vi "UHR-Fleezers Control (host) - Lorentz v5.vi"() -> ()   [LabVIEW 2014] (continued)
  n60 = Bundle("New Image"=w49, "New Image"=w48, "New Image"=w31, "New Image"=w47, "New Image"=w46) -> (w45:T34)  [unwired: 1 in]
  n61 = xnode "Open FPGA VI Reference"("resource name"=T27 "RIO0") -> ("FPGA VI Reference Out"=w26:T35, "error out"=w25:errorcluster)  [unwired: 1 in]
  n62 = xnode "Invoke Method"("FPGA VI Reference In"=w26, "error in"=w25) -> ("FPGA VI Reference Out"=w6:T35, "error out"=→"FPGA error out":errorcluster)
  n63 = Subtract(x=w4, y="Maximum Delta\n(MHz)") -> (x-y=w2:dbl)
  n64 = Bundle By Name(cluster=T23 {"Minimum"=60.0, "Maximum"=90.0, "Increment"=1.0} ("Min Max Inc"), "Minimum"=w2, "Maximum"=w4) -> (w1:T23)
  n65 = node-c288() -> (w52:T36)  [unwired: 4 in]
  n66 = timed-loop "Run Scripts, including: stage motion" {
    tunnel: w55 -> [w218]
    tunnel: w9 -> [w219]
    tunnel: [w219] -> w54
    tunnel: [w218] -> w53
    timing: w52 -> [_]
    timing-out: [_] -> w51
    tunnel: w43 -> [w217]
    tunnel: w44 -> [w216]
    tunnel: w39 -> [w213]
    tunnel: w38 -> [w212]
    tunnel: w37 -> [w214]
    tunnel: w36 -> [w215]
    tunnel: w28 -> [w211]
    tunnel: w21 -> [w210]
    tunnel: w8 -> [w209]
    tunnel: w7 -> [w208]
    stop <- w220 stop-if-true
    n67 = node-c288() -> ()  [unwired: 1 in, 1 out]
    n68 = event shown="[17] \"Got Bead 1\": Value Change" {
      selector: _ -> [_ _ _ _ _ _ _ _ _ _ _ _ _ _ _ _ _ _ _ _ _ _ _ _ _ _ _ _]
      dyn-events: _ -> [_ _ _ _ _ _ _ _ _ _ _ _ _ _ _ _ _ _ _ _ _ _ _ _ _ _ _ _]
      timeout: _ -> [_ _ _ _ _ _ _ _ _ _ _ _ _ _ _ _ _ _ _ _ _ _ _ _ _ _ _ _]
      tunnel: ["Set Position" "Move to Position" _ _ _ _ _ _ "Read Harvard" _ _ _ _ _ _ _ _ "Got Bead 1" "Force FB Data\nScript" _ "Got Bead 2" _ "Take Stepping Data" _ "Take Detection Laser\nImage" _ _ _] -> _
      tunnel: [_ _ _ _ _ _ _ _ _ _ _ _ _ _ _ _ _ _ _ _ _ _ _ _ _ _ w1147 _] -> w220
      tunnel: w218 -> [w239 w247 w260 w290 _ _ _ _ _ w427 w461 w487 w519 w608 w637 w769 w796 _ w838 _ _ _ _ _ _ _ _ _]
      tunnel: w219 -> [w240 w248 w261 w291 _ _ _ _ _ w428 w462 w488 w520 w609 w638 w770 w797 _ w839 _ _ _ _ _ _ _ _ _]
      tunnel: w217 -> [_ _ _ _ _ _ _ _ w412 _ _ _ _ _ _ _ _ _ _ _ _ _ _ _ _ _ _ _]
      tunnel: w216 -> [_ _ _ _ _ _ _ _ w411 _ _ _ _ _ _ _ _ _ _ _ _ _ _ _ _ _ _ _]
      tunnel: w215 -> [_ _ _ _ _ _ _ _ _ _ _ _ _ _ _ _ _ _ _ _ _ _ _ _ _ _ _ _]
      tunnel: w214 -> [_ _ _ _ _ _ _ _ _ _ _ _ _ _ _ _ _ _ _ _ _ _ _ _ _ _ _ _]
      tunnel: w213 -> [_ _ _ _ _ _ _ _ _ _ _ _ _ _ _ _ _ _ _ _ _ _ _ _ _ _ _ _]
      tunnel: w212 -> [_ _ _ _ _ _ _ _ _ _ _ _ _ _ _ _ _ _ _ _ _ _ _ _ _ _ _ _]
      tunnel: w211 -> [_ _ _ _ w318 w325 w353 w372 _ _ _ _ _ _ _ _ _ _ _ _ _ _ _ _ _ _ w1146 _]
      tunnel: w210 -> [_ _ _ _ _ _ _ _ _ _ _ _ _ _ _ _ _ _ _ _ _ _ _ _ _ w1013 _ _]
      tunnel: w209 -> [_ _ _ _ _ _ _ _ _ _ _ _ _ _ _ _ _ _ _ _ _ _ _ _ _ _ _ w1157]
      tunnel: w208 -> [_ _ _ _ _ _ _ _ _ _ _ _ _ _ _ _ _ _ _ _ _ _ _ _ _ _ _ w1152]
      tunnel: [_ _ _ _ _ _ _ _ _ _ _ _ _ _ _ _ _ _ _ _ _ "Get New Beads" _ _ _ _ _ _] -> _
      event "Set Position", "Set Position 2", "Set Position 3", "Set Position 4", "Set Position 5", "Set Position 1", "Set Position 6": Value Change {
        n69 = event-data() -> ()  [unwired: 1 in, 5 out]
        n70 = Build Array("Set Position 1", "Set Position 2", "Set Position 3", "Set Position 4", "Set Position 5", "Set Position 6") -> (w238:bool[])
        n71 = Boolean Array To Number(Boolean array=w238) -> (number=w237:u32)
        n72 = Logarithm Base 2(1:w237) -> (0:w229:dbl)
        n73 = call "Read Stage Position.vi"("error in"=w239, "VISA resource name in"=w240) -> ("Current Position"=w244:cluster{dbl, dbl, dbl}, "error out"=w243:errorcluster)  [unwired: 2 out]
        n74 = Decrement(x="Position") -> (x-1=w227:dbl)
        n75 = Greater Or Equal?(x=w229, y=0.0) -> (x >= y?=w230:bool)
        n76 = Cluster To Array(cluster=w244) -> (array=w241:dbl[])
        n77 = local write "Stage Control Serial Error"(w243) -> ()
        n78 = Select(t=w229, s=w230, f=w227) -> (s? t:f=w226:dbl)
        n79 = Increment(x=w226) -> (x+1=w225:dbl)
        n80 = Build Array (concatenate)(w225, w241) -> (w224:dbl[])
        n81 = Replace Array Subset(array="Saved Stage Positions", new element=w224, index (row)=w226) -> (w242:dbl[][])  [unwired: 1 in]
        n82 = local write "Saved Stage Positions"(w242) -> ()
      }
      event "Move to Position": Value Change {
        n83 = event-data() -> ()  [unwired: 1 in, 5 out]
        n84 = flat-sequence {
          tunnel: w248 -> [w252]
          tunnel: w247 -> [w251]
          frame #0 {
            n85 = local read "Saved Stage Positions"() -> (w254:dbl[][])
            n86 = local read "Position"() -> (w253:dbl)
            n87 = local write "Stage Moving"(TRUE ("Stage Moving")) -> ()
            n88 = call "move to saved stage position.vi"("error in"=w251, "Stage VISA resource name in"=w252, "Position"=w253, "Saved Stage Positions"=w254) -> ("error out"=w250:errorcluster)  [unwired: 1 out]
            n89 = local write "Stage Control Serial Error"(w250) -> ()
          }
          frame #1 {
            n90 = call <vilib>:"Beep.vi"() -> ()  [unwired: 3 in, 9 out]
            n91 = local write "Stage Moving"(FALSE ("Stage Moving")) -> ()
          }
        }
      }
      event "Move Cap. 1 (DNA Bottom)": Value Change {
        n92 = event-data() -> ()  [unwired: 1 in, 5 out]
        n93 = local write "Move Cap. 1 (DNA Bottom)"(FALSE ("Move Cap. 1 (DNA Right)")) -> ()
        n94 = flat-sequence {
          tunnel: w260 -> [w263]
          tunnel: w261 -> [w264]
          tunnel: [w264] -> w258
          tunnel: [w263] -> w257
          tunnel: w258 -> [w266]
          tunnel: w257 -> [w265]
          frame #0 {
            n95 = property on="Sample Channel\nFlow" class="Bool (strict)"("Val(Sgnl)"="Cap 1 Samp Flow ON") -> ()  [unwired: 2 in, 2 out]
          }
          frame #1 {
            n96 = local read "Saved Stage Positions"() -> (w276:dbl[][])
            n97 = local write "Stage Moving"(TRUE ("Stage Moving")) -> ()
            n98 = Array Subset(array=w276, index (row)=0 ("index"), length (row)=1 ("length"), index (col)=1 ("index"), length (col)=3 ("length")) -> (w273:dbl[][])
            n99 = Reshape Array(w273, 3 ("dimension size")) -> (w271:dbl[])
            n100 = Array To Cluster(array=w271) -> (cluster=w270:cluster{"[0]":dbl, "[1]":dbl, "[2]":dbl})
            n101 = call "Set Stage Position.vi"("Position"=w270, "error in"=w265, "VISA resource name in"=w266) -> ("error out"=w269:errorcluster)  [unwired: 2 out]
            n102 = local write "Stage Control Serial Error"(w269) -> ()
          }
          frame #2 {
            n103 = local write "Stage Moving"(FALSE ("Stage Moving")) -> ()
            n104 = case shown="True" "Cap 1 Flow ON" {
              frame False {
              }
              frame True {
                n105 = property on="Inject Pump 1" class="Bool (strict)"("Val(Sgnl)"=TRUE ("Value (Signaling)")) -> ()  [unwired: 2 in, 2 out]
              }
            }
            n106 = call <vilib>:"Beep.vi"() -> ()  [unwired: 3 in, 9 out]
          }
          frame #3 {
            n107 = property on="Sample Channel\nFlow" class="Bool (strict)"("Val(Sgnl)"=FALSE ("Value (Signaling)")) -> ()  [unwired: 2 in, 2 out]
            n108 = local read "Cap. 2 BD T1?\n(ADig T1, DNA T2)"() -> (w283:bool)
            n109 = case shown="True" w283 {
              tunnel: "Cap 1 T ON" -> [w285 w286]
              frame False {
                n110 = property on="Trap 1 (ON/OFF)" class="Bool (strict)"("Val(Sgnl)"=w285) -> ()  [unwired: 2 in, 2 out]
              }
              frame True {
                n111 = property on="Trap 2 (ON/OFF)" class="Bool (strict)"("Val(Sgnl)"=w286) -> ()  [unwired: 2 in, 2 out]
              }
            }
            n112 = property on="Got Bead 2" class="Bool"("Key Focus"=TRUE) -> ()  [unwired: 2 in, 2 out]
          }
        }
      }
      event "Move Cap. 2 (ADig Top)": Value Change {
        n113 = event-data() -> ()  [unwired: 1 in, 5 out]
        n114 = local write "Move Cap. 2 (ADig Top)"(FALSE ("Move Cap. 2 (ADig Left)")) -> ()
        n115 = flat-sequence {
          tunnel: w290 -> [w293]
          tunnel: w291 -> [w294]
          tunnel: [w294] -> w288
          tunnel: [w293] -> w287
          tunnel: w288 -> [w297]
          tunnel: w287 -> [w296]
          frame #0 {
            n116 = property on="Sample Channel\nFlow" class="Bool (strict)"("Val(Sgnl)"="Cap 2 Samp Flow ON") -> ()  [unwired: 2 in, 2 out]
          }
          frame #1 {
            w295 = FALSE ("Value (Signaling)")
            n117 = local read "Saved Stage Positions"() -> (w307:dbl[][])
            n118 = local write "Stage Moving"(TRUE ("Stage Moving")) -> ()
            n119 = Array Subset(array=w307, index (row)=1 ("index"), length (row)=1 ("length"), index (col)=1 ("index"), length (col)=3 ("length")) -> (w304:dbl[][])
            n120 = Reshape Array(w304, 3 ("dimension size")) -> (w302:dbl[])
            n121 = property on="Trap 1 (ON/OFF)" class="Bool (strict)"("Val(Sgnl)"=w295) -> ()  [unwired: 2 in, 2 out]
            n122 = property on="Trap 1 (ON/OFF)" class="Bool (strict)"("Val(Sgnl)"=w295) -> ()  [unwired: 2 in, 2 out]
            n123 = Array To Cluster(array=w302) -> (cluster=w301:cluster{"[0]":dbl, "[1]":dbl, "[2]":dbl})
            n124 = call "Set Stage Position.vi"("Position"=w301, "error in"=w296, "VISA resource name in"=w297) -> ("error out"=w300:errorcluster)  [unwired: 2 out]
            n125 = local write "Stage Control Serial Error"(w300) -> ()
          }
          frame #2 {
            n126 = local write "Stage Moving"(FALSE ("Stage Moving")) -> ()
            n127 = call <vilib>:"Beep.vi"() -> ()  [unwired: 3 in, 9 out]
            n128 = case shown="True" "Cap 2 Flow ON" {
              frame False {
              }
              frame True {
                n129 = property on="Inject Pump 3" class="Bool (strict)"("Val(Sgnl)"=TRUE ("Value (Signaling)")) -> ()  [unwired: 2 in, 2 out]
              }
            }
          }
          frame #3 {
            n130 = property on="Sample Channel\nFlow" class="Bool (strict)"("Val(Sgnl)"=FALSE ("Value (Signaling)")) -> ()  [unwired: 2 in, 2 out]
            n131 = case shown="False" "Cap. 2 BD T1?\n(ADig T1, DNA T2)" {
              tunnel: "Cap 2 T ON" -> [w316 w317]
              frame False {
                n132 = property on="Trap 2 (ON/OFF)" class="Bool (strict)"("Val(Sgnl)"=w316) -> ()  [unwired: 2 in, 2 out]
              }
              frame True {
                n133 = property on="Trap 1 (ON/OFF)" class="Bool (strict)"("Val(Sgnl)"=w317) -> ()  [unwired: 2 in, 2 out]
              }
            }
            n134 = property on="Got Bead 1" class="Bool"("Key Focus"=TRUE) -> ()  [unwired: 2 in, 2 out]
          }
        }
      }
      event "Send string\nto Blue Laser": Value Change {
        n135 = event-data() -> ()  [unwired: 1 in, 5 out]
        n136 = flat-sequence {
          tunnel: w318 -> [w319]
          frame #0 {
            n137 = call "serial write macro.vi"("String"="command string", "Delay (ms)"="Delay (ms)", "VISA resource name"=w319) -> ("read buffer"=→"read blue buffer":string, "error out"=→"Blue Error Out":errorcluster)  [unwired: 1 out]
            "command string sent" <- "command string"
          }
          frame #1 {
            n138 = local write "Send string\nto Blue Laser"(FALSE ("Send string")) -> ()
          }
        }
      }
      event "Get Blue Laser State": Value Change {
        n139 = event-data() -> ()  [unwired: 1 in, 5 out]
        n140 = local read "Delay (ms)"() -> (w326:i32)
        n141 = flat-sequence {
          tunnel: w326 -> [w334]
          tunnel: w325 -> [w337]
          tunnel: [w335] -> w330
          tunnel: [w334] -> w329
          tunnel: [w344] -> w328
          tunnel: [w341] -> w327
          tunnel: w330 -> [w342]
          tunnel: w329 -> [w341]
          tunnel: w328 -> [w350]
          tunnel: w327 -> [w348]
          frame #0 {
            w332 = "l?"
            n142 = local write "command string sent"(w332) -> ()
            n143 = call "serial write macro.vi"("String"=w332, "Delay (ms)"=w334, "VISA resource name"=w337) -> ("read buffer"=w333:string, "VISA resource name out"=w335:refnum<visa-resource-name>)  [unwired: 1 out]
            n144 = Decimal String To Number(string=w333) -> (number=w336:i32)  [unwired: 2 in, 1 out]
            n145 = Not Equal To 0?(x=w336) -> (x != 0?=→"Laser On":bool)
            n146 = local write "read blue buffer"(w333) -> ()
          }
          frame #1 {
            w339 = "games?" ("String")
            n147 = local write "command string sent"(w339) -> ()
            n148 = call "serial write macro.vi"("String"=w339, "Delay (ms)"=w341, "VISA resource name"=w342) -> ("read buffer"=w340:string, "VISA resource name out"=w344:refnum<visa-resource-name>)  [unwired: 1 out]
            n149 = Decimal String To Number(string=w340) -> (number=w343:i32)  [unwired: 2 in, 1 out]
            n150 = local write "read blue buffer"(w340) -> ()
            n151 = Not Equal To 0?(x=w343) -> (x != 0?=→"Analog Modulation":bool)
          }
          frame #2 {
            w346 = "gdmes?" ("String")
            n152 = local write "command string sent"(w346) -> ()
            n153 = call "serial write macro.vi"("String"=w346, "Delay (ms)"=w348, "VISA resource name"=w350) -> ("read buffer"=w347:string)  [unwired: 2 out]
            n154 = Decimal String To Number(string=w347) -> (number=w349:i32)  [unwired: 2 in, 1 out]
            n155 = Not Equal To 0?(x=w349) -> (x != 0?=→"Digital Modulation":bool)
            n156 = local write "read blue buffer"(w347) -> ()
          }
          frame #3 {
            n157 = local write "Get Blue Laser State"(FALSE) -> ()
          }
        }
      }
      event "Blue Laser Power (mW)\n(Constant Power Mode)", "Blue Laser Modulation\nPower (mW)": Value Change {
        n158 = event-data() -> ()  [unwired: 1 in, 5 out]
        n159 = flat-sequence {
          tunnel: w353 -> [w359]
          tunnel: [w357] -> w352
          tunnel: w352 -> [w366]
          frame #0 {
            n160 = local read "Delay (ms)"() -> (w358:i32)
            n161 = Concatenate Strings("slmp " ("string"), "Blue Laser Modulation\nPower (mW)") -> (w354:string)
            n162 = call "serial write macro.vi"("String"=w354, "Delay (ms)"=w358, "VISA resource name"=w359) -> ("read buffer"=w355:string, "error out"=w356:errorcluster, "VISA resource name out"=w357:refnum<visa-resource-name>)
            n163 = local write "command string sent"(w354) -> ()
            n164 = local write "read blue buffer"(w355) -> ()
            n165 = local write "Blue Error Out"(w356) -> ()
          }
          frame #1 {
            n166 = local read "Delay (ms)"() -> (w365:i32)
            n167 = Concatenate Strings("p " ("string"), "Blue Laser Power (mW)\n(Constant Power Mode)") -> (w362:string)
            n168 = call "serial write macro.vi"("String"=w362, "Delay (ms)"=w365, "VISA resource name"=w366) -> ("read buffer"=w363:string, "error out"=w364:errorcluster)  [unwired: 1 out]
            n169 = local write "command string sent"(w362) -> ()
            n170 = local write "read blue buffer"(w363) -> ()
            n171 = local write "Blue Error Out"(w364) -> ()
          }
        }
      }
      event "Laser interlacing mode", "Blue Laser Modulation Mode", "Blue Laser ON": Value Change {
        n172 = event-data() -> ()  [unwired: 1 in, 5 out]
        n173 = flat-sequence {
          tunnel: w372 -> [w377]
          tunnel: [w376] -> w369
          tunnel: [w382] -> w371
          tunnel: w369 -> [w385]
          tunnel: w371 -> [w397]
          tunnel: [w391] -> w370
          tunnel: w370 -> [w404]
          frame #0 {
            n174 = local read "Blue Laser ON"() -> (w374:bool)
            n175 = local read "Delay (ms)"() -> (w375:i32)
            n176 = case shown="False" w374 {
              tunnel: ["l0" "l1"] -> w373
              frame False {
              }
              frame True {
              }
            }
            n177 = call "serial write macro.vi"("String"=w373, "Delay (ms)"=w375, "VISA resource name"=w377) -> ("error out"=w378:errorcluster, "VISA resource name out"=w376:refnum<visa-resource-name>)  [unwired: 1 out]
            n178 = local write "Blue Error Out"(w378) -> ()
          }
          frame #1 {
            n179 = local read "Laser interlacing mode"() -> (w387:enum32{"Laser ON", "Laser OFF", "Interlace"})
            n180 = case shown="\"Laser ON\"" w387 {
              tunnel: ["cp" "em" "l0"] -> w381
              frame "Laser ON" {
              }
              frame "Interlace" {
              }
              frame "Laser OFF", Default {
              }
            }
            n181 = local read "Delay (ms)"() -> (w386:i32)
            n182 = call "serial write macro.vi"("String"=w381, "Delay (ms)"=w386, "VISA resource name"=w385) -> ("read buffer"=w383:string, "error out"=w384:errorcluster, "VISA resource name out"=w382:refnum<visa-resource-name>)
            n183 = local write "command string sent"(w381) -> ()
            n184 = local write "read blue buffer"(w383) -> ()
            n185 = local write "Blue Error Out"(w384) -> ()
          }
          frame #2 {
            n186 = case shown="\"Analog Modulation\"" "Blue Laser Modulation Mode" {
              tunnel: ["sdmes 0" "sdmes 1" "sdmes 1"] -> w392
              frame "Analog Modulation" {
              }
              frame "Digital + Analog Modulation" {
              }
              frame "Digital Modulation", Default {
              }
            }
            n187 = local read "Delay (ms)"() -> (w395:i32)
            n188 = call "serial write macro.vi"("String"=w392, "Delay (ms)"=w395, "VISA resource name"=w397) -> ("read buffer"=w393:string, "error out"=w394:errorcluster, "VISA resource name out"=w391:refnum<visa-resource-name>)
            n189 = local write "command string sent"(w392) -> ()
            n190 = local write "read blue buffer"(w393) -> ()
            n191 = local write "Blue Error Out"(w394) -> ()
          }
          frame #3 {
            n192 = local read "Blue Laser Modulation Mode"() -> (w406:string)
            n193 = case shown="\"Digital Modulation\", Default" w406 {
              tunnel: ["sames 1" "sames 1" "sames 0"] -> w402
              frame "Analog Modulation" {
              }
              frame "Digital + Analog Modulation" {
              }
              frame "Digital Modulation", Default {
              }
            }
            n194 = local read "Delay (ms)"() -> (w405:i32)
            n195 = local write "command string sent"(w402) -> ()
            n196 = call "serial write macro.vi"("String"=w402, "Delay (ms)"=w405, "VISA resource name"=w404) -> ("read buffer"=w403:string, "error out"=w401:errorcluster)  [unwired: 1 out]
            n197 = local write "read blue buffer"(w403) -> ()
            n198 = local write "Blue Error Out"(w401) -> ()
          }
        }
      }
      event "Read Harvard": Value Change {
        n199 = event-data() -> ()  [unwired: 1 in, 5 out]
        n200 = Concatenate Strings("write buffer", "\r") -> (w414:string)
        n201 = VISA Write(VISA resource name=w412, write buffer=w414, error in (no error)=w411) -> (VISA resource name out=w423:refnum<visa-resource-name>, error out=w422:errorcluster)  [unwired: 1 out]
        n202 = stacked-sequence {
          tunnel: [w426] -> w421
          tunnel: w423 -> [w426]
          tunnel: w422 -> [w425]
          tunnel: [w425] -> w416
          frame #0 {
            n203 = Wait (ms)(milliseconds to wait=50) -> ()  [unwired: 1 out]
          }
        }
        n204 = property class="Instr"(reference=w421, error in=w416) -> (reference out=w420:refnum<visa-resource-name>, error out=w418:errorcluster, "Serial Settings:Number of Bytes at Serial Port"=w419:u32)
        "Serial Settings:Number of Bytes at Serial Port" <- w419
        n205 = VISA Read(VISA resource name=w420, byte count=w419, error in (no error)=w418) -> (read buffer=w417:string)  [unwired: 3 out]
        "read buffer" <- w417
        n206 = Fract/Exp String To Number(string=w417) -> ()  [unwired: 5 out]
      }
      event "+z", "-z": Value Change {
        n207 = event-data() -> ()  [unwired: 1 in, 5 out]
        n208 = flat-sequence {
          tunnel: w427 -> [w449]
          tunnel: w428 -> [w429]
          frame #0 {
            n209 = call "Read Stage Position.vi"("error in"=w449, "VISA resource name in"=w429) -> ("Current Position"=w434:cluster{dbl, dbl, dbl}, "error out"=w447:errorcluster, "VISA resource name out"=w448:refnum<visa-resource-name>)  [unwired: 1 out]
            n210 = local read "Saved Stage Positions"() -> (w458:dbl[][])
            n211 = Divide(x="z nudge increment (um)", y=1000.0) -> (x/y=w446:dbl)
            n212 = Boolean To (0,1)(Boolean="+z") -> (0, 1=w438:i16)
            n213 = Boolean To (0,1)(Boolean="-z") -> (0, 1=w439:i16)
            n214 = Array Subset(array=w458, index (row)=1 ("index"), length (row)=1 ("length"), index (col)=1 ("index"), length (col)=3 ("length")) -> (w455:dbl[][])
            n215 = Multiply(x=w438, y=w446) -> (x*y=w442:dbl)
            n216 = Multiply(x=w439, y=w446) -> (x*y=w440:dbl)
            n217 = Unbundle(w434) -> (w432:dbl, w431:dbl, w435:dbl)
            n218 = Negate(x=w440) -> (-x=w441:dbl)
            n219 = Reshape Array(w455, 3 ("dimension size")) -> (w453:dbl[])
            n220 = Add(x=w442, y=w441) -> (x+y=w443:dbl)
            n221 = Array To Cluster(array=w453) -> ()  [unwired: 1 out]
            n222 = Add(x=w443, y=w435) -> (x+y=w433:dbl)
            n223 = Bundle(cluster=w434, w432, w431, w433) -> (w430:cluster{dbl, dbl, dbl})
            n224 = call "Set Stage Position.vi"("Position"=w430, "error in"=w447, "VISA resource name in"=w448) -> ("error out"=w452:errorcluster)  [unwired: 2 out]
            n225 = local write "Stage Moving"(TRUE ("Stage Moving")) -> ()
            n226 = local write "Stage Control Serial Error"(w452) -> ()
          }
          frame #1 {
            n227 = local write "Stage Moving"(FALSE ("Stage Moving")) -> ()
          }
        }
      }
      event "-y", "+y": Value Change {
        n228 = event-data() -> ()  [unwired: 1 in, 5 out]
        n229 = flat-sequence {
          tunnel: w461 -> [w485]
          tunnel: w462 -> [w468]
          frame #0 {
            n230 = call "Read Stage Position.vi"("error in"=w485, "VISA resource name in"=w468) -> ("Current Position"=w471:cluster{dbl, dbl, dbl}, "error out"=w483:errorcluster, "VISA resource name out"=w484:refnum<visa-resource-name>)  [unwired: 1 out]
            n231 = Divide(x="y nudge increment (um", y=1000.0) -> (x/y=w482:dbl)
            n232 = Boolean To (0,1)(Boolean="+y") -> (0, 1=w474:i16)
            n233 = Boolean To (0,1)(Boolean="-y") -> (0, 1=w475:i16)
            n234 = Multiply(x=w474, y=w482) -> (x*y=w478:dbl)
            n235 = Multiply(x=w475, y=w482) -> (x*y=w476:dbl)
            n236 = Unbundle(w471) -> (w470:dbl, w465:dbl, w467:dbl)
            n237 = Negate(x=w476) -> (-x=w477:dbl)
            n238 = Add(x=w478, y=w477) -> (x+y=w479:dbl)
            n239 = Add(x=w479, y=w465) -> (x+y=w466:dbl)
            n240 = Bundle(cluster=w471, w470, w466, w467) -> (w469:cluster{dbl, dbl, dbl})
            n241 = call "Set Stage Position.vi"("Position"=w469, "error in"=w483, "VISA resource name in"=w484) -> ("error out"=w464:errorcluster)  [unwired: 2 out]
            n242 = local write "Stage Control Serial Error"(w464) -> ()
            n243 = local write "Stage Moving"(TRUE ("Stage Moving")) -> ()
          }
          frame #1 {
            n244 = local write "Stage Moving"(FALSE ("Stage Moving")) -> ()
          }
        }
      }
      event "-x", "+x": Value Change {
        n245 = event-data() -> ()  [unwired: 1 in, 5 out]
        n246 = flat-sequence {
          tunnel: w487 -> [w511]
          tunnel: w488 -> [w495]
          frame #0 {
            n247 = call "Read Stage Position.vi"("error in"=w511, "VISA resource name in"=w495) -> ("Current Position"=w497:cluster{dbl, dbl, dbl}, "error out"=w509:errorcluster, "VISA resource name out"=w510:refnum<visa-resource-name>)  [unwired: 1 out]
            n248 = Divide(x="x nudge increment (um)", y=1000.0) -> (x/y=w508:dbl)
            n249 = Boolean To (0,1)(Boolean="+x") -> (0, 1=w500:i16)
            n250 = Boolean To (0,1)(Boolean="-x") -> (0, 1=w501:i16)
            n251 = Multiply(x=w500, y=w508) -> (x*y=w504:dbl)
            n252 = Multiply(x=w501, y=w508) -> (x*y=w502:dbl)
            n253 = Unbundle(w497) -> (w489:dbl, w491:dbl, w494:dbl)
            n254 = Negate(x=w502) -> (-x=w503:dbl)
            n255 = Add(x=w504, y=w503) -> (x+y=w505:dbl)
            n256 = Add(x=w505, y=w489) -> (x+y=w490:dbl)
            n257 = Bundle(cluster=w497, w490, w491, w494) -> (w496:cluster{dbl, dbl, dbl})
            n258 = call "Set Stage Position.vi"("Position"=w496, "error in"=w509, "VISA resource name in"=w510) -> ("error out"=w492:errorcluster)  [unwired: 2 out]
            n259 = local write "Stage Control Serial Error"(w492) -> ()
            n260 = local write "Stage Moving"(TRUE ("Stage Moving")) -> ()
          }
          frame #1 {
            n261 = local write "Stage Moving"(FALSE ("Stage Moving")) -> ()
          }
        }
      }
      event "Cal/Data Acq. Spot": Value Change {
        # "Disabled by Ronen - we have our own way of controlling the location of calibration."
        n262 = event-data() -> ()  [unwired: 1 in, 5 out]
        n263 = flat-sequence {
          tunnel: w519 -> [w523]
          tunnel: w520 -> [w524]
          tunnel: [w524] -> w516
          tunnel: [w523] -> w515
          tunnel: w516 -> [w527]
          tunnel: w515 -> [w526]
          tunnel: ["Cal @ (MHz)"] -> w513
          tunnel: [w535] -> w517
          tunnel: w513 -> [w535]
          tunnel: w517 -> [w547]
          tunnel: ["W/ Offset 1"] -> w514
          tunnel: w517 -> [w568]
          tunnel: w514 -> [w566]
          frame #0 {
            n264 = property on="Sample Channel\nFlow" class="Bool (strict)"("Val(Sgnl)"="Daq spot flow on") -> ()  [unwired: 2 in, 2 out]
            n265 = Wait (ms)(milliseconds to wait=u32 250) -> ()  [unwired: 1 out]
          }
          frame #1 {
            n266 = disable-structure shown="Disabled" {
              disable-tunnel: w527 -> [w532 _]
              disable-tunnel: w526 -> [w531 _]
              frame Disabled {
                n267 = local read "Saved Stage Positions"() -> (w529:dbl[][])
                n268 = call "move to saved stage position.vi"("error in"=w531, "Stage VISA resource name in"=w532, "Position"="Cal Stage Position", "Saved Stage Positions"=w529) -> ("error out"=w530:errorcluster)  [unwired: 1 out]
                n269 = local write "Stage Control Serial Error"(w530) -> ()
              }
              frame Enabled {
              }
            }
            n270 = property on="Trap Delta (MHz)" class="DigNum (strict)"("Val(Sgnl)"="Cal @ (MHz)") -> ()  [unwired: 2 in, 2 out]
            n271 = local write "Stage Moving"(TRUE ("Stage Moving")) -> ()
          }
          frame #2 {
            n272 = local write "Stage Moving"(FALSE ("Stage Moving")) -> ()
            n273 = property on="Sample Channel\nFlow" class="Bool (strict)"("Val(Sgnl)"="Flow ON during cal?") -> ()  [unwired: 2 in, 2 out]
            n274 = call <vilib>:"Beep.vi"() -> ()  [unwired: 3 in, 9 out]
          }
          frame #3 {
            n275 = Wait (ms)(milliseconds to wait=u32 1000) -> ()  [unwired: 1 out]
          }
          frame #4 {
            n276 = case shown="True" "Active cal after cal?" {
              frame False {
              }
              frame True {
                n277 = local write "Active Cal"(TRUE ("Active Cal")) -> ()
                n278 = Wait (ms)(milliseconds to wait=u32 8000) -> ()  [unwired: 1 out]
              }
            }
          }
          frame #5 {
            n279 = property on="Save Calibration" class="Bool (strict)"("Val(Sgnl)"=TRUE ("Value (Signaling)")) -> ()  [unwired: 2 in, 2 out]
          }
          frame #6 {
            n280 = Wait (ms)(milliseconds to wait=u32 2000) -> ()  [unwired: 1 out]
          }
          frame #7 {
            # "Check to see if \nsaving done"
            n281 = while {
              stop <- w543 stop-if-true
              n282 = local read "Saving..."() -> (w544:bool)
              n283 = Wait (ms)(milliseconds to wait=u32 100) -> ()  [unwired: 1 out]
              n284 = Not(x=w544) -> (.not. x?=w543:bool)
            }
          }
          frame #8 {
            n285 = case shown="True" "W/ Offset 1" {
              tunnel: w547 -> [_ w548]
              frame False {
              }
              frame True {
                n286 = stacked-sequence {
                  tunnel: w548 -> [_ _ _ _ _ _ _ w565]
                  frame #0 {
                    n287 = property on="Trap Delta (MHz)" class="DigNum (strict)"("Val(Sgnl)"="Offset 1 Start (MHz)") -> ()  [unwired: 2 in, 2 out]
                    n288 = Replace Array Subset(array=u32[] [0] ("Index Values"), new element="Offset 1 Set", index=0) -> (w550:u32[])
                    n289 = property on="Saved AOD Raster Scan Parameter Sets" class="Arr (strict)"("Index Values"=w550) -> ()  [unwired: 2 in, 2 out]
                    n290 = property on="manual raster set" class="Ring (strict)"("Value"="Offset 1 Set") -> ()  [unwired: 2 in, 2 out]
                  }
                  frame #1 {
                    n291 = Wait (ms)(milliseconds to wait=u32 200) -> ()  [unwired: 1 out]
                  }
                  frame #2 {
                    n292 = property on="Load parameters" class="Bool (strict)"("Val(Sgnl)"=TRUE ("Value (Signaling)")) -> ()  [unwired: 2 in, 2 out]
                  }
                  frame #3 {
                    n293 = Wait (ms)(milliseconds to wait=u32 200) -> ()  [unwired: 1 out]
                  }
                  frame #4 {
                    n294 = property on="Trap Raster Scan" class="Bool (strict)"("Val(Sgnl)"=TRUE ("Value (Signaling)")) -> ()  [unwired: 2 in, 2 out]
                  }
                  frame #5 {
                    n295 = Wait (ms)(milliseconds to wait=u32 2000) -> ()  [unwired: 1 out]
                  }
                  frame #6 {
                    n296 = while {
                      stop <- w562 stop-if-true
                      n297 = local read "Raster Scanning..."() -> (w564:bool)
                      n298 = local read "Saving..."() -> (w560:bool)
                      n299 = Wait (ms)(milliseconds to wait=u32 100) -> ()  [unwired: 1 out]
                      n300 = Not(x=w560) -> (.not. x?=w559:bool)
                      n301 = Not(x=w564) -> (.not. x?=w561:bool)
                      n302 = And(x=w561, y=w559) -> (x .and. y?=w562:bool)
                    }
                  }
                  frame #7 {
                    n303 = property on="Trap Delta (MHz)" class="DigNum (strict)"("Val(Sgnl)"=w565) -> ()  [unwired: 2 in, 2 out]
                  }
                }
              }
            }
          }
          frame #9 {
            n304 = local read "Save ave N"() -> (w567:dbl)
            n305 = case shown="True" "W/ Offset 2" {
              tunnel: w568 -> [_ w575]
              tunnel: w567 -> [_ w574]
              tunnel: w566 -> [w570 _]
              frame False {
                n306 = case shown="False" w570 {
                  frame False {
                    n307 = Multiply(x="Cal read wait (s)", y=u32 1000 ("milliseconds to wait")) -> (x*y=w572:u32)
                    n308 = Wait (ms)(milliseconds to wait=w572) -> ()  [unwired: 1 out]
                  }
                  frame True {
                  }
                }
              }
              frame True {
                n309 = stacked-sequence {
                  tunnel: w575 -> [_ _ _ _ _ _ _ _ _ w596 _ _]
                  tunnel: w574 -> [_ _ _ _ _ _ _ _ _ w594 _ _]
                  frame #0 {
                    n310 = property on="Save ave N" class="DigNum (strict)"("Val(Sgnl)"=1.0 ("Value (Signaling)")) -> ()  [unwired: 2 in, 2 out]
                  }
                  frame #1 {
                    n311 = Wait (ms)(milliseconds to wait=u32 500) -> ()  [unwired: 1 out]
                  }
                  frame #2 {
                    n312 = property on="Trap Delta (MHz)" class="DigNum (strict)"("Val(Sgnl)"="Offset 2 Start (MHz)") -> ()  [unwired: 2 in, 2 out]
                    n313 = Replace Array Subset(array=u32[] [0] ("Index Values"), new element="Offset 2 Set", index=0) -> (w580:u32[])
                    n314 = property on="Saved AOD Raster Scan Parameter Sets" class="Arr (strict)"("Index Values"=w580) -> ()  [unwired: 2 in, 2 out]
                  }
                  frame #3 {
                    n315 = Wait (ms)(milliseconds to wait=u32 500) -> ()  [unwired: 1 out]
                  }
                  frame #4 {
                    n316 = property on="Load parameters" class="Bool (strict)"("Val(Sgnl)"=TRUE ("Value (Signaling)")) -> ()  [unwired: 2 in, 2 out]
                  }
                  frame #5 {
                    n317 = Wait (ms)(milliseconds to wait=u32 500) -> ()  [unwired: 1 out]
                  }
                  frame #6 {
                    n318 = property on="Trap Raster Scan" class="Bool (strict)"("Val(Sgnl)"=TRUE ("Value (Signaling)")) -> ()  [unwired: 2 in, 2 out]
                  }
                  frame #7 {
                    n319 = Wait (ms)(milliseconds to wait=u32 2000) -> ()  [unwired: 1 out]
                  }
                  frame #8 {
                    n320 = while {
                      stop <- w589 stop-if-true
                      n321 = local read "Raster Scanning..."() -> (w592:bool)
                      n322 = local read "Saving..."() -> (w590:bool)
                      n323 = Wait (ms)(milliseconds to wait=u32 100) -> ()  [unwired: 1 out]
                      n324 = Not(x=w590) -> (.not. x?=w588:bool)
                      n325 = Not(x=w592) -> (.not. x?=w591:bool)
                      n326 = And(x=w591, y=w588) -> (x .and. y?=w589:bool)
                    }
                  }
                  frame #9 {
                    n327 = property on="Trap Delta (MHz)" class="DigNum (strict)"("Val(Sgnl)"=w596) -> ()  [unwired: 2 in, 2 out]
                    n328 = property on="Saved AOD Raster Scan Parameter Sets" class="Arr (strict)"("Index Values"=u32[] [0]) -> ()  [unwired: 2 in, 2 out]
                    n329 = property on="Save ave N" class="DigNum (strict)"("Val(Sgnl)"=w594) -> ()  [unwired: 2 in, 2 out]
                  }
                  frame #10 {
                    n330 = Wait (ms)(milliseconds to wait=u32 500) -> ()  [unwired: 1 out]
                  }
                  frame #11 {
                    n331 = property on="Load parameters" class="Bool (strict)"("Val(Sgnl)"=TRUE ("Value (Signaling)")) -> ()  [unwired: 2 in, 2 out]
                  }
                }
              }
            }
          }
          frame #10 {
            # "Added by Ronen for flow calibration"
            n332 = case shown="True" "Flow based calibration?" {
              frame False {
              }
              frame True {
                n333 = stacked-sequence {
                  frame #0 {
                    n334 = local write "Flow Cal"(TRUE) -> ()
                  }
                  frame #1 {
                  }
                  frame #2 {
                    n335 = Wait (ms)(milliseconds to wait=u32 8000) -> ()  [unwired: 1 out]
                  }
                }
              }
            }
          }
          frame #11 {
            n336 = property on="Read Cal" class="Bool (strict)"("Val(Sgnl)"=TRUE ("Value (Signaling)")) -> ()  [unwired: 2 in, 2 out]
          }
          frame #12 {
            n337 = Wait (ms)(milliseconds to wait=u32 1000) -> ()  [unwired: 1 out]
          }
          frame #13 {
            n338 = property on="Fish for Tether" class="Bool (strict)"("Val(Sgnl)"="Fish after cal?") -> ()  [unwired: 2 in, 2 out]
          }
        }
        n339 = local write "Cal/Data Acq. Spot"(FALSE ("Cal/Data Acq. Spot")) -> ()
      }
      event "Dump Beads": Value Change {
        n340 = event-data() -> ()  [unwired: 1 in, 5 out]
        n341 = flat-sequence {
          tunnel: ["Dump spot flow on?"] -> w605
          tunnel: [w616] -> w606
          tunnel: w605 -> [w616]
          tunnel: w609 -> [w621]
          tunnel: w608 -> [w620]
          tunnel: [w618] -> w607
          tunnel: w606 -> [w618]
          tunnel: w607 -> [w631]
          frame #0 {
            w610 = FALSE ("Value (Signaling)")
            n342 = local read "Saving..."() -> (w612:bool)
            n343 = local write "Dump Beads"(FALSE ("Dump Beads")) -> ()
            n344 = property on="Inject Pump 3" class="Bool (strict)"("Val(Sgnl)"=w610) -> ()  [unwired: 2 in, 2 out]
            n345 = property on="Inject Pump 1" class="Bool (strict)"("Val(Sgnl)"=w610) -> ()  [unwired: 2 in, 2 out]
            n346 = local write "Stop Saving"(w612) -> ()
          }
          frame #1 {
            w613 = FALSE ("Fl. Triggered...")
            n347 = case shown="True" "Dump spot flow on?" {
              frame False {
              }
              frame True {
                n348 = property on="Sample Channel\nFlow" class="Bool (strict)"("Val(Sgnl)"=TRUE ("Stage Moving")) -> ()  [unwired: 2 in, 2 out]
              }
            }
            n349 = local write "Fl. Triggered..."(w613) -> ()
            n350 = local write "Tether"(w613) -> ()
            n351 = property on="Green Laser ON" class="Bool (strict)"("Val(Sgnl)"=w613) -> ()  [unwired: 2 in, 2 out]
            n352 = property on="Trap Pos. FB ON" class="Bool (strict)"("Val(Sgnl)"=w613) -> ()  [unwired: 2 in, 2 out]
            n353 = property on="Trap Trig. Fl." class="Bool (strict)"("Val(Sgnl)"=w613) -> ()  [unwired: 2 in, 2 out]
            n354 = property on="Fl. Triggered..." class="Bool (strict)"("Val(Sgnl)"=w613) -> ()  [unwired: 2 in, 2 out]
            n355 = property on="Dip for Protein" class="Bool (strict)"("Val(Sgnl)"=w613) -> ()  [unwired: 2 in, 2 out]
            n356 = property on="Pause dwell" class="Bool (strict)"("Val(Sgnl)"=w613) -> ()  [unwired: 2 in, 2 out]
          }
          frame #2 {
            n357 = property on="Trap Pos. FB Offset Factor" class="DigNum (strict)"("Val(Sgnl)"=i64 0 ("Value (Signaling)")) -> ()  [unwired: 2 in, 2 out]
          }
          frame #3 {
            n358 = local read "Saved Stage Positions"() -> (w622:dbl[][])
            n359 = local write "Stage Moving"(TRUE ("Stage Moving")) -> ()
            n360 = Array Subset(array=w622, index (row)=3 ("index"), length (row)=1 ("length"), index (col)=1 ("index"), length (col)=3 ("length")) -> (w627:dbl[][])
            n361 = Reshape Array(w627, 3 ("dimension size")) -> (w625:dbl[])
            n362 = Array To Cluster(array=w625) -> (cluster=w624:cluster{"[0]":dbl, "[1]":dbl, "[2]":dbl})
            n363 = call "Set Stage Position.vi"("Position"=w624, "error in"=w620, "VISA resource name in"=w621) -> ()  [unwired: 3 out]
          }
          frame #4 {
            w632 = FALSE ("Value (Signaling)")
            n364 = case shown="True" w631 {
              frame False {
              }
              frame True {
                n365 = property on="Sample Channel\nFlow" class="Bool (strict)"("Val(Sgnl)"=FALSE ("Stage Moving")) -> ()  [unwired: 2 in, 2 out]
              }
            }
            n366 = property on="Trap 1 (ON/OFF)" class="Bool (strict)"("Val(Sgnl)"=w632) -> ()  [unwired: 2 in, 2 out]
            n367 = property on="Trap 2 (ON/OFF)" class="Bool (strict)"("Val(Sgnl)"=w632) -> ()  [unwired: 2 in, 2 out]
            n368 = call <vilib>:"Beep.vi"() -> ()  [unwired: 3 in, 9 out]
          }
          frame #5 {
            n369 = property on="Move Cap. 2 (ADig Top)" class="Bool (strict)"("Val(Sgnl)"=TRUE ("Value (Signaling)")) -> ()  [unwired: 2 in, 2 out]
            n370 = property on="Tab Control" class="TabCtl (strict)"("Val(Sgnl)"=T39."Status" ("Value (Signaling)")) -> ()  [unwired: 2 in, 2 out]
          }
        }
      }
      event "Dip for Protein": Value Change {
        n371 = event-data() -> ()  [unwired: 1 in, 5 out]
        n372 = case shown="True" "Dip for Protein" {
          tunnel: w638 -> [_ w640]
          tunnel: w637 -> [_ w639]
          frame False {
          }
          frame True {
            n373 = while {
              tunnel: w640 -> [w651]
              tunnel: w639 -> [w650]
              i -> [w645]
              stop <- w647 stop-if-true
              n374 = Increment(x=w645) -> (x+1=→"Dip #":i32)
              n375 = flat-sequence {
                tunnel: w650 -> [w662]
                tunnel: w651 -> [w663]
                tunnel: [w663] -> w655
                tunnel: [w662] -> w654
                tunnel: [w656] -> w641
                tunnel: [w668] -> w649
                tunnel: [w669] -> w648
                tunnel: w655 -> [w670]
                tunnel: w654 -> [w671]
                tunnel: [w666] -> w642
                tunnel: w641 -> [w666]
                tunnel: [w679] -> w653
                tunnel: w649 -> [w679]
                tunnel: [w678] -> w652
                tunnel: w648 -> [w678]
                tunnel: [w675] -> w646
                tunnel: [w674] -> w643
                tunnel: w642 -> [w674]
                tunnel: w652 -> [w699]
                tunnel: w653 -> [w700]
                tunnel: w646 -> [w701]
                tunnel: w643 -> [w698]
                tunnel: [w757] -> w647
                frame #0 {
                  n376 = local read "Trap Pos. FB ON"() -> (w656:bool)
                  n377 = Compound Arithmetic op=AND("Flow ON\nduring dip?", "FB OFF when \nflow ON", w656) -> (w657:bool)
                  n378 = case shown="True" "Move trap \nbefore dip move?" {
                    frame False {
                    }
                    frame True {
                      n379 = property on="Trap Delta (MHz)" class="DigNum (strict)"("Val(Sgnl)"="Dipping Delta (MHz)") -> ()  [unwired: 2 in, 2 out]
                    }
                  }
                  n380 = property on="Green Laser ON" class="Bool (strict)"("Val(Sgnl)"="Green ON\nbefore dip?") -> ()  [unwired: 2 in, 2 out]
                  n381 = property on="Sample Channel\nFlow" class="Bool (strict)"("Val(Sgnl)"="Flow ON\nduring dip?") -> ()  [unwired: 2 in, 2 out]
                  n382 = case shown="True" w657 {
                    frame False {
                    }
                    frame True {
                      n383 = property on="Trap Pos. FB ON" class="Bool (strict)"("Val(Sgnl)"=FALSE ("Value (Signaling)")) -> ()  [unwired: 2 in, 2 out]
                    }
                  }
                }
                frame #1 {
                  n384 = local read "Saved Stage Positions"() -> (w673:dbl[][])
                  n385 = local write "Cancel dwell"(FALSE ("Cancel dwell")) -> ()
                  n386 = call "move to saved stage position.vi"("error in"=w671, "Stage VISA resource name in"=w670, "Position"="Dip Stage \nPosition", "Saved Stage Positions"=w673) -> ("VISA resource name out"=w668:refnum<visa-resource-name>, "error out"=w669:errorcluster)
                }
                frame #2 {
                  n387 = node-c288() -> (w677:T36)  [unwired: 4 in]
                  n388 = timed-loop {
                    timing: w677 -> [_]
                    timing-out: [_] -> w676
                    tunnel: [w683] -> w675
                    i -> [w680]
                    stop <- w684 stop-if-true
                    n389 = node-c288() -> ()  [unwired: 1 in, 1 out]
                    n390 = Greater Or Equal?(x=w680, y="Dip Duration (s)") -> (x >= y?=w692:bool)
                    n391 = local read "Dip for Protein"() -> (w685:bool)
                    n392 = local read "Dump Beads"() -> (w682:bool)
                    n393 = local read "Cancel dwell"() -> (w691:bool)
                    n394 = local read "Pause dwell"() -> (w688:bool)
                    n395 = Not(x=w685) -> (.not. x?=w690:bool)
                    n396 = Compound Arithmetic op=OR(w691, w692, w690) -> (w689:bool)
                    n397 = Select(t=FALSE, s=w688, f=w689) -> (s? t:f=w686:bool)
                    n398 = Not(x=w682) -> (.not. x?=w681:bool)
                    n399 = node-c288() -> ()  [unwired: 1 in, 1 out]
                    n400 = And(x=w685, y=w681) -> (x .and. y?=w683:bool)
                    n401 = Or(x=w686, y=w682) -> (x .or. y?=w684:bool)
                    "Dip Time (s)" <- w680
                  }
                  n402 = node-c288(w676) -> ()  [unwired: 1 out]
                }
                frame #3 {
                  n403 = case shown="True" w701 {
                    tunnel: w700 -> [_ w706]
                    tunnel: w699 -> [_ w705]
                    tunnel: w698 -> [_ w702]
                    frame False {
                    }
                    frame True {
                      n404 = flat-sequence {
                        tunnel: w705 -> [w710]
                        tunnel: w706 -> [w711]
                        tunnel: [w711] -> w704
                        tunnel: [w710] -> w703
                        tunnel: w702 -> [w707]
                        tunnel: w704 -> [w721]
                        tunnel: w703 -> [w720]
                        tunnel: w702 -> [w729]
                        frame #0 {
                          n405 = local read "Sample Channel\nFlow"() -> (w709:bool)
                          n406 = case shown="True" w709 {
                            tunnel: "Flow ON \nduring return\nfrom dip?" -> [w712 w715]
                            tunnel: w707 -> [_ w714]
                            frame False {
                              n407 = case shown="True" w712 {
                                frame False {
                                }
                                frame True {
                                n408 = property on="Sample Channel\nFlow" class="Bool (strict)"("Val(Sgnl)"=TRUE ("Value (Signaling)")) -> ()  [unwired: 2 in, 2 out]
                                }
                              }
                            }
                            frame True {
                              n409 = case shown="False" w715 {
                                tunnel: w714 -> [w716 _]
                                frame False {
                                n410 = property on="Trap Pos. FB ON" class="Bool (strict)"("Val(Sgnl)"=w716) -> ()  [unwired: 2 in, 2 out]
                                n411 = property on="Sample Channel\nFlow" class="Bool (strict)"("Val(Sgnl)"=FALSE ("Value (Signaling)")) -> ()  [unwired: 2 in, 2 out]
                                }
                                frame True {
                                }
                              }
                            }
                          }
                        }
                        frame #1 {
                          # "For turning on green laser before stage reaches lower spot"
                          n412 = case shown="True" "Green ON\nafter start\nreturn?" {
                            frame False {
                            }
                            frame True {
                              n413 = flat-sequence {
                                frame #0 {
                                n414 = Multiply(x="Green delay after \nstart return (s)", y=1000.0) -> (x*y=w726:dbl)
                                n415 = Wait (ms)(milliseconds to wait=w726) -> ()  [unwired: 1 out]
                                }
                                frame #1 {
                                n416 = property on="Green Laser ON" class="Bool (strict)"("Val(Sgnl)"=TRUE ("Value (Signaling)")) -> ()  [unwired: 2 in, 2 out]
                                }
                              }
                            }
                          }
                          n417 = local read "Saved Stage Positions"() -> (w724:dbl[][])
                          n418 = local write "Cancel dwell"(FALSE ("Cancel dwell")) -> ()
                          n419 = call "move to saved stage position.vi"("error in"=w720, "Stage VISA resource name in"=w721, "Position"="Return Stage \nPosition", "Saved Stage Positions"=w724) -> ("error out"=w722:errorcluster)  [unwired: 1 out]
                          n420 = local write "Stage Control Serial Error"(w722) -> ()
                        }
                        frame #2 {
                          n421 = property on="Trap Pos. FB ON" class="Bool (strict)"("Val(Sgnl)"=w729) -> ()  [unwired: 2 in, 2 out]
                          n422 = case shown="True" "Green ON \nafter return?" {
                            frame False {
                            }
                            frame True {
                              n423 = property on="Green Laser ON" class="Bool (strict)"("Val(Sgnl)"=TRUE ("Value (Signaling)")) -> ()  [unwired: 2 in, 2 out]
                            }
                          }
                          n424 = case shown="True" "Move trap after return?" {
                            frame False {
                            }
                            frame True {
                              n425 = property on="Trap Delta (MHz)" class="DigNum (strict)"("Val(Sgnl)"="Dip Trap Delta 2 (MHz)") -> ()  [unwired: 2 in, 2 out]
                            }
                          }
                          n426 = case shown="True" "Save data after return?" {
                            frame False {
                            }
                            frame True {
                              n427 = property on="Start Saving" class="Bool (strict)"("Val(Sgnl)"=TRUE ("Value (Signaling)")) -> ()  [unwired: 2 in, 2 out]
                            }
                          }
                          n428 = property on="Sample Channel\nFlow" class="Bool (strict)"("Val(Sgnl)"="Flow ON\nduring daq?") -> ()  [unwired: 2 in, 2 out]
                        }
                        frame #3 {
                          n429 = node-c288() -> (w738:T36)  [unwired: 4 in]
                          n430 = timed-loop {
                            timing: w738 -> [_]
                            timing-out: [_] -> w737
                            i -> [w739]
                            stop <- w741 stop-if-true
                            n431 = node-c288() -> ()  [unwired: 1 in, 1 out]
                            n432 = local read "Dump Beads"() -> (w740:bool)
                            n433 = Greater Or Equal?(x=w739, y="Dwell Duration (s)") -> (x >= y?=w746:bool)
                            n434 = local read "Dip for Protein"() -> (w743:bool)
                            n435 = Not(x=w743) -> (.not. x?=w742:bool)
                            n436 = Compound Arithmetic op=OR(w746, "Cancel dwell", w742) -> (w745:bool)
                            n437 = node-c288() -> ()  [unwired: 1 in, 1 out]
                            n438 = Select(t=FALSE, s="Pause dwell", f=w745) -> (s? t:f=w748:bool)
                            n439 = Or(x=w748, y=w740) -> (x .or. y?=w741:bool)
                            "Dwell Time (s)" <- w739
                          }
                          n440 = node-c288(w737) -> ()  [unwired: 1 out]
                        }
                      }
                    }
                  }
                }
                frame #4 {
                  n441 = local read "Dip for Protein"() -> (w758:bool)
                  n442 = local read "Dump Beads"() -> (w755:bool)
                  n443 = local write "Cancel dwell"(FALSE ("Cancel dwell")) -> ()
                  n444 = Not(x=w758) -> (.not. x?=w759:bool)
                  n445 = Not(x="Cont. Repeat Dipping?") -> (.not. x?=w761:bool)
                  n446 = Compound Arithmetic op=OR(w759, w761, w755) -> (w757:bool)
                }
              }
            }
          }
        }
      }
      event "Profile": Value Change {
        n447 = event-data() -> ()  [unwired: 1 in, 5 out]
        n448 = flat-sequence {
          tunnel: w770 -> [w773]
          tunnel: w769 -> [w781]
          tunnel: [w775] -> w768
          tunnel: [w774] -> w767
          tunnel: [w772] -> w765
          tunnel: [w771] -> w762
          tunnel: w768 -> [w788]
          tunnel: w767 -> [w787]
          tunnel: [w785] -> w766
          tunnel: w765 -> [w786]
          tunnel: [w784] -> w764
          tunnel: [w783] -> w763
          tunnel: w762 -> [w783]
          tunnel: w766 -> [w792]
          tunnel: w764 -> [w791]
          tunnel: w763 -> [w790]
          frame #0 {
            n449 = call "Read Stage Position.vi"("error in"=w781, "VISA resource name in"=w773) -> ("Current Position"=w771:cluster{dbl, dbl, dbl}, "error out"=w774:errorcluster, "VISA resource name out"=w772:refnum<visa-resource-name>)  [unwired: 1 out]
